vi "ReplayAuto.vi"(11 "file path (use dialog)":path=path "/home/lvuser/natinst/bin/data/RecordedPaths/RecordedAuto.4153") -> ()   [LabVIEW 2023]
uses:
  Swerve Setpoints.ctl
  Swerve Operations.ctl
  <vilib>/Rock Robotics/WPI/ThirdParty/JAS_Junk/TrajLib/TypeDef/CHASSIS_SPEEDS.ctl
  <vilib>/Rock Robotics/WPI/ThirdParty/JAS_Junk/TrajLib/Trajectory_Library.lvlib
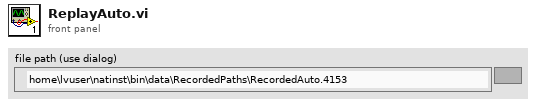
[diagram p1: front panel]
types:
  T1 = enum16{"open", "replace", "create", "open or create", "replace or create", "replace or create with confirmation"}
  T2 = typedef "Swerve Operations.ctl" = enum16{"Reserve", "Read Current", "Immediate", "Joystick Drive"}
  T3 = typedef "Swerve Setpoints.ctl" = cluster{"Operation":T2, "CHASSIS":T4}
  T4 = typedef "Trajectory_Library.lvlib/CHASSIS_SPEEDS.ctl" = cluster{"vX":dbl, "vY":dbl, "vOmega":dbl}
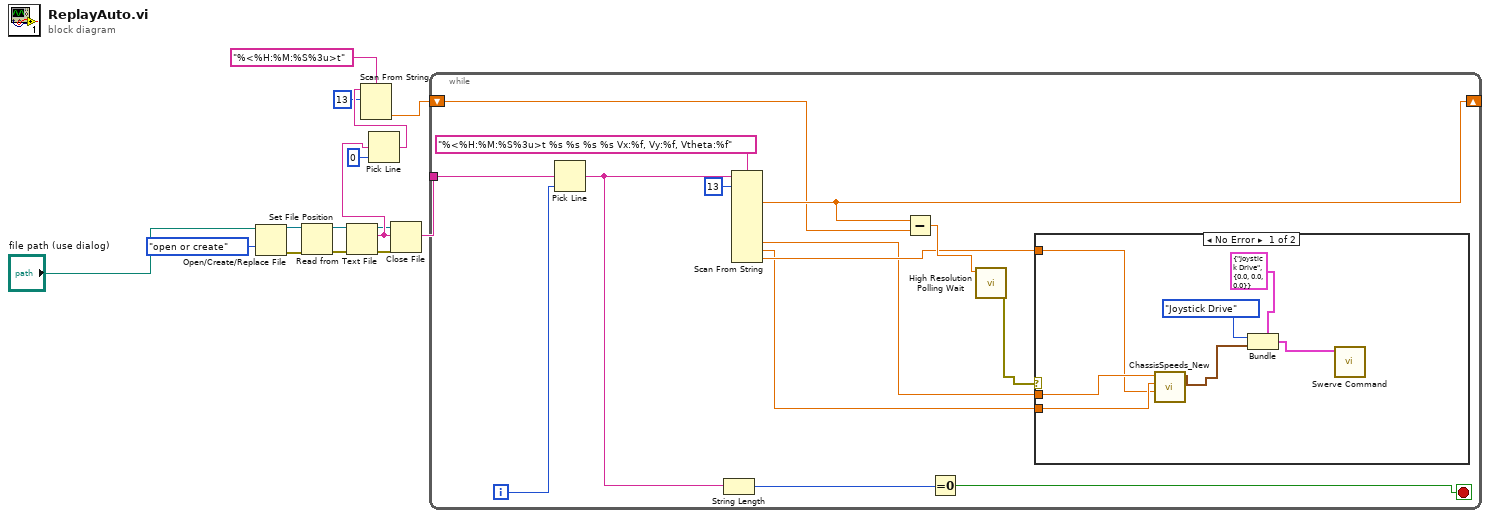
[diagram p0: block diagram]
diagram:
  n1 = Open/Create/Replace File(file path (use dialog)="file path (use dialog)", operation (0:open)=T1."open or create") -> (refnum out=w13:refnum<file>, error out=w12:errorcluster)  [unwired: 4 in, 1 out]
  n2 = Set File Position(refnum=w13, error in=w12) -> (refnum out=w10:refnum<file>, error out=w11:errorcluster)  [unwired: 2 in]
  n3 = Read from Text File(file (use dialog)=w10, error in=w11) -> (refnum out=w1:refnum<file>, text=w8:string, error out=w2:errorcluster)  [unwired: 2 in, 1 out]
  n4 = Pick Line(multi-line string=w8, line index=0) -> (output string=w6:string)  [unwired: 1 in]
  n5 = Scan From String(format string="%<%H:%M:%S%3u>t", input string=w6, initial scan location=u32 13) -> (output 1=w5:dbl)  [unwired: 2 in, 3 out]
  n6 = Close File(refnum=w1, error in=w2) -> ()  [unwired: 2 out]
  n7 = while {
    tunnel: w8 -> [w25]
    shift-right: [w22] -> _
    shift-left: w5 -> [w21]
    i -> [w24]
    stop <- w27 stop-if-true
    n8 = Pick Line(multi-line string=w25, line index=w24) -> (output string=w18:string)  [unwired: 1 in]
    n9 = String Length(string=w18) -> (length=w26:i32)
    n10 = Scan From String(format string="%<%H:%M:%S%3u>t %s %s %s %s Vx:%f, Vy:%f, Vtheta:%f", input string=w18, initial scan location=u32 13) -> (output 1=w22:dbl, output 6=w16:dbl, output 7=w15:dbl, output 8=w17:dbl)  [unwired: 13 in, 3 out]
    n11 = Subtract(x=w22, y=w21) -> (x-y=w20:dbl)
    n12 = Equal To 0?(x=w26) -> (x = 0?=w27:bool)
    n13 = call <vilib>:"High Resolution Polling Wait.vi"("seconds to wait"=w20) -> ("error out"=w19:errorcluster)  [unwired: 10 in]
    n14 = case shown="No Error" w19 {
      tunnel: w16 -> [w31 _]
      tunnel: w15 -> [w30 _]
      tunnel: w17 -> [w29 _]
      frame No Error {
        n15 = call <vilib>:"ChassisSpeeds_New.vi"("vAngular"=w29, "vY"=w30, "vX"=w31) -> ("CHASSIS"=w32:T4)  [unwired: 8 in]
        n16 = Bundle(cluster=T3 {"Operation"=enum."Joystick Drive", "CHASSIS"={"vX"=0.0, "vY"=0.0, "vOmega"=0.0}} ("SubSystem Data"), "Operation"=Swerve_Operations."Joystick Drive", "CHASSIS"=w32) -> (w34:T3)
        n17 = call "Swerve Command.vi"("SubSystem Data"=w34) -> ()  [unwired: 10 in, 1 out]
      }
      frame Error {
      }
    }
  }
